vi "Anritsu1a_MT8852B_YYLL_InitialSetting.vi"(11 "YTESTER测试数据":T1) -> (3 "YTESTER结论":T2)   [LabVIEW 2017]
doc: "VIDescription="
uses:
  YtCommon.lvlibp/yt`Step StepBaseInput.ctl
  YtCommon.lvlibp/yt`Step StepResult.ctl
  YtCommon.lvlibp/yt`Step TestData.ctl
  YtCommon.lvlibp/yt`Step System Queue.ctl
  YtCommon.lvlibp
panel:
  out "Show":bool
  out "view send":string
  out "read buffer":string
  in  "YTESTER开放参数":T4={"YTESTER_BaseInput"={"isTest"=TRUE, "isSkip"=FALSE, "StepName"="AnritsuMT8852B初始化", "OnPass"=enum."Next", "OnFail"=enum."Terminate", "ReTestNumber"=0.0}, "VISA resource name"="", "EUT搜索时间[5,60]"=10, "低频线损dB[-40,0]"=-0.1, "中频线损dB[-40,0]"=-0.1, "高频线损dB[-40,0]"=-0.1, "功率输出测试-包类型"=enum."DH1", "单隙灵敏度测试-Tx发射功率dBm[-90,0]"=-70.0, "单隙灵敏度测试-包数量[1,10000]"=600}
  # "initialSetting"
  # "MT8852B"
  # "Anritsu"
  # "YYLL"
  # "MT8852B"
  # "Anritsu"
  # "YYLL"
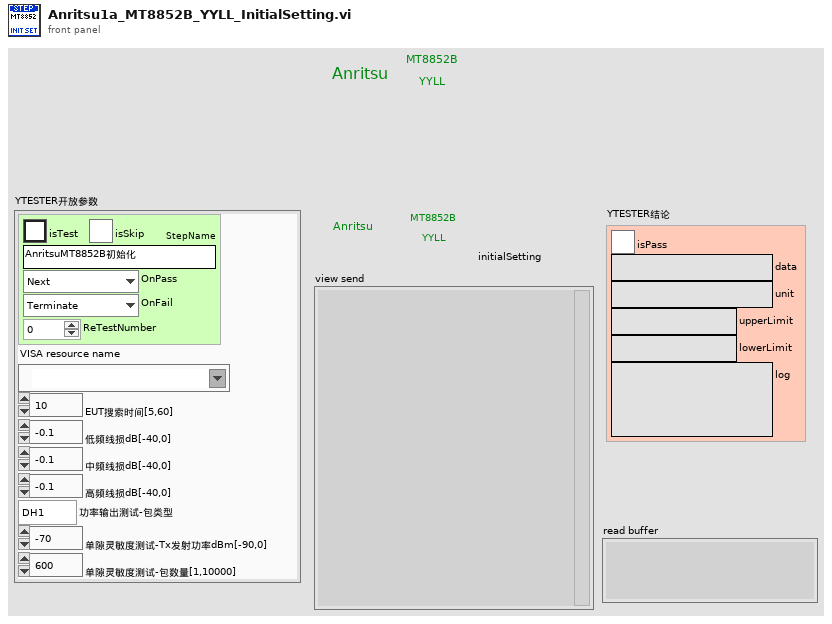
[diagram p1: front panel]
types:
  T1 = typedef "YtCommon.lvlibp/yt`Step TestData.ctl" = cluster{"Socket(From1)":i32, "SN":refnum<notifier>, "StopFlagRef":refnum<notifier>, "YT System Queue":refnum<queue>}
  T2 = typedef "YtCommon.lvlibp/yt`Step StepResult.ctl" = cluster{"isPass":bool, "data":string, "unit":string, "upperLimit":string, "lowerLimit":string, "log":string}
  T3 = typedef "YtCommon.lvlibp/yt`Step StepBaseInput.ctl" = cluster{"isTest":bool, "isSkip":bool, "StepName":string, "OnPass":enum16{"Next", "ToOVER", "Terminate"}, "OnFail":enum16{"Next", "ToOVER", "Terminate"}, "ReTestNumber":dbl}
  T4 = cluster{"YTESTER_BaseInput":T3, "VISA resource name":refnum<visa-resource-name>, "EUT搜索时间[5,60]":u32, "低频线损dB[-40,0]":dbl, "中频线损dB[-40,0]":dbl, "高频线损dB[-40,0]":dbl, "功率输出测试-包类型":enum16{"DH1", "DH3", "DH5", "LONG"}, "单隙灵敏度测试-Tx发射功率dBm[-90,0]":dbl, "单隙灵敏度测试-包数量[1,10000]":u32}
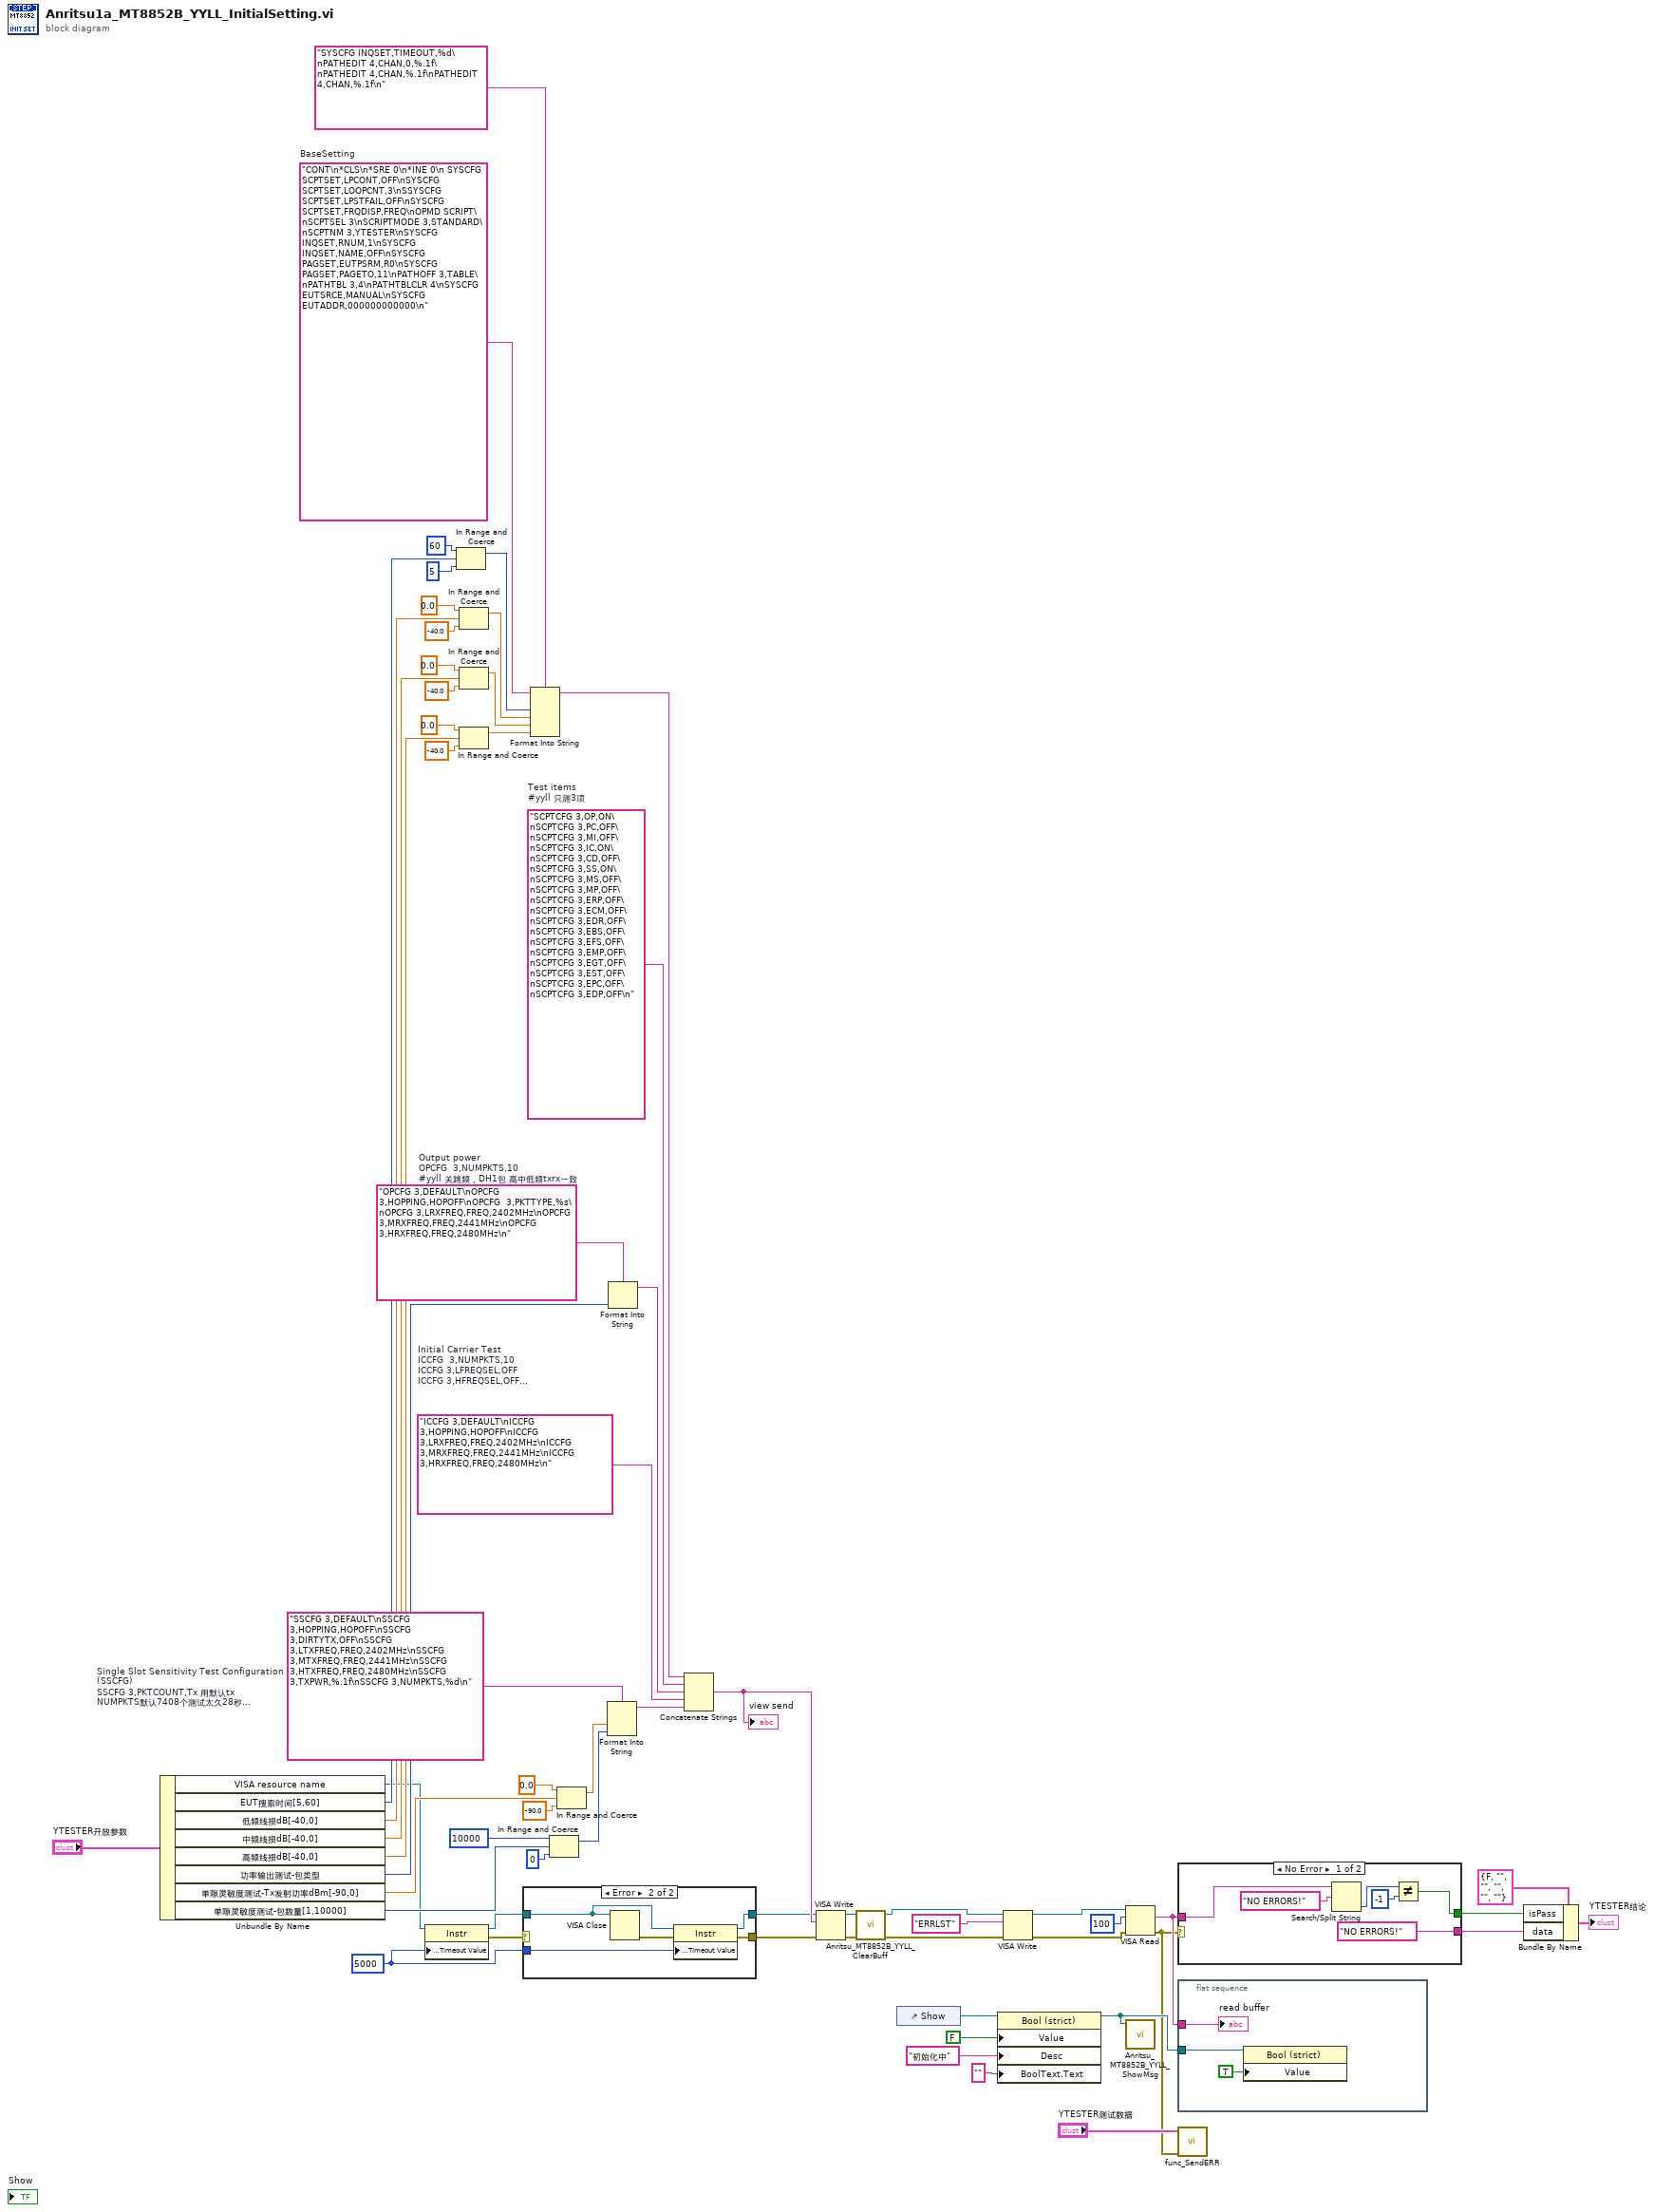
[diagram p0: block diagram]
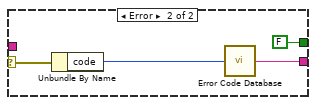
[diagram p3: hidden frame]
diagram:
  w6 = u32 5000 ("General Settings:Timeout Value")
  w21 = "SSCFG 3,DEFAULT\nSSCFG 3,HOPPING,HOPOFF\nSSCFG 3,DIRTYTX,OFF\nSSCFG 3,LTXFREQ,FREQ,2402MHz\nSSCFG 3,MTXFREQ,FREQ,2441MHz\nSSCFG 3,HTXFREQ,FREQ,2480MHz\nSSCFG 3,TXPWR,%.1f\nSSCFG 3,NUMPKTS,%d\n"  # Single Slot Sensitivity Test Configuration (SSCFG)  SSCFG 3,PKTCOUNT,Tx 用默认tx NUMPKTS默认7408个测试太久28秒 控制在600个包吧 #yyll
  w55 = "ICCFG 3,DEFAULT\nICCFG 3,HOPPING,HOPOFF\nICCFG 3,LRXFREQ,FREQ,2402MHz\nICCFG 3,MRXFREQ,FREQ,2441MHz\nICCFG 3,HRXFREQ,FREQ,2480MHz\n"  # Initial Carrier Test  ICCFG  3,NUMPKTS,10 ICCFG 3,LFREQSEL,OFF ICCFG 3,HFREQSEL,OFF #yyll 这里只测中频，关跳频，中频txrx一致 还是都测吧
  w28 = "OPCFG 3,DEFAULT\nOPCFG 3,HOPPING,HOPOFF\nOPCFG  3,PKTTYPE,%s\nOPCFG 3,LRXFREQ,FREQ,2402MHz\nOPCFG 3,MRXFREQ,FREQ,2441MHz\nOPCFG 3,HRXFREQ,FREQ,2480MHz\n"  # Output power OPCFG  3,NUMPKTS,10 #yyll 关跳频，DH1包 高中低频txrx一致
  w60 = "SCPTCFG 3,OP,ON\nSCPTCFG 3,PC,OFF\nSCPTCFG 3,MI,OFF\nSCPTCFG 3,IC,ON\nSCPTCFG 3,CD,OFF\nSCPTCFG 3,SS,ON\nSCPTCFG 3,MS,OFF\nSCPTCFG 3,MP,OFF\nSCPTCFG 3,ERP,OFF\nSCPTCFG 3,ECM,OFF\nSCPTCFG 3,EDR,OFF\nSCPTCFG 3,EBS,OFF\nSCPTCFG 3,EFS,OFF\nSCPTCFG 3,EMP,OFF\nSCPTCFG 3,EGT,OFF\nSCPTCFG 3,EST,OFF\nSCPTCFG 3,EPC,OFF\nSCPTCFG 3,EDP,OFF\n"  # Test items #yyll 只测3项
  w35 = "CONT\n*CLS\n*SRE 0\n*INE 0\n SYSCFG SCPTSET,LPCONT,OFF\nSYSCFG SCPTSET,LOOPCNT,3\nSSYSCFG SCPTSET,LPSTFAIL,OFF\nSYSCFG SCPTSET,FRQDISP,FREQ\nOPMD SCRIPT\nSCPTSEL 3\nSCRIPTMODE 3,STANDARD\nSCPTNM 3,YTESTER\nSYSCFG INQSET,RNUM,1\nSYSCFG INQSET,NAME,OFF\nSYSCFG PAGSET,EUTPSRM,R0\nSYSCFG PAGSET,PAGETO,11\nPATHOFF 3,TABLE\nPATHTBL 3,4\nPATHTBLCLR 4\nSYSCFG EUTSRCE,MANUAL\nSYSCFG EUTADDR,000000000000\n"  # BaseSetting
  n1 = Unbundle By Name("YTESTER开放参数") -> ("VISA resource name"=w5:refnum<visa-resource-name>, "EUT搜索时间[5,60]"=w49:u32, "低频线损dB[-40,0]"=w39:dbl, "中频线损dB[-40,0]"=w38:dbl, "高频线损dB[-40,0]"=w37:dbl, "功率输出测试-包类型"=w30:enum16{"DH1", "DH3", "DH5", "LONG"}, "单隙灵敏度测试-Tx发射功率dBm[-90,0]"=w25:dbl, "单隙灵敏度测试-包数量[1,10000]"=w22:u32)
  n2 = property class="Instr"(reference=w5, "General Settings:Timeout Value"=w6) -> (reference out=w7:refnum<visa-resource-name>, error out=w8:errorcluster)  [unwired: 1 in]
  n3 = In Range and Coerce(upper limit=u32 60, x=w49, lower limit=u32 5) -> (coerced(x)=w46:u32)  [unwired: 1 out]
  n4 = In Range and Coerce(upper limit=0.0, x=w39, lower limit=-40.0) -> (coerced(x)=w34:dbl)  [unwired: 1 out]
  n5 = In Range and Coerce(upper limit=0.0, x=w38, lower limit=-40.0) -> (coerced(x)=w33:dbl)  [unwired: 1 out]
  n6 = In Range and Coerce(upper limit=0.0, x=w37, lower limit=-40.0) -> (coerced(x)=w32:dbl)  [unwired: 1 out]
  n7 = case shown="Error" w8 {
    selector: w8 -> [w63 _]
    tunnel: w7 -> [w64 w69]
    tunnel: w6 -> [_ w67]
    tunnel: [w63 w66] -> w3
    tunnel: [w64 w65] -> w4
    frame No Error {
    }
    frame Error {
      n8 = VISA Close(VISA resource name=w69) -> (error out=w68:errorcluster)  [unwired: 1 in]
      n9 = property class="Instr"(reference=w69, error in=w68, "General Settings:Timeout Value"=w67) -> (reference out=w65:refnum<visa-resource-name>, error out=w66:errorcluster)
    }
  }
  n10 = Format Into String(format string="SYSCFG INQSET,TIMEOUT,%d\nPATHEDIT 4,CHAN,0,%.1f\nPATHEDIT 4,CHAN,%.1f\nPATHEDIT 4,CHAN,%.1f\n", initial string=w35, w46, w34, w33, w32) -> (resulting string=w31:string)  [unwired: 1 in, 1 out]
  n11 = In Range and Coerce(upper limit=u32 10000, x=w22, lower limit=u32 0) -> (coerced(x)=w19:u32)  [unwired: 1 out]
  n12 = In Range and Coerce(upper limit=0.0, x=w25, lower limit=-90.0) -> (coerced(x)=w20:dbl)  [unwired: 1 out]
  n13 = Format Into String(format string=w21, w20, w19) -> (resulting string=w16:string)  [unwired: 2 in, 1 out]
  n14 = Format Into String(format string=w28, w30) -> (resulting string=w29:string)  [unwired: 2 in, 1 out]
  n15 = Concatenate Strings(w31, w60, w29, w55, w16) -> (w17:string)
  "view send" <- w17
  n16 = VISA Write(VISA resource name=w4, write buffer=w17, error in (no error)=w3) -> (VISA resource name out=w54:refnum<visa-resource-name>, error out=w52:errorcluster)  [unwired: 1 out]
  n17 = call "Anritsu_MT8852B_YYLL_ClearBuff.vi"("error IO"=w52, "VISA resource name"=w54) -> ("error IO 2"=w51:errorcluster, "VISA resource name 2"=w53:refnum<visa-resource-name>)  [unwired: 7 in, 1 out]
  n18 = control-ref of="Show"() -> (w15:refnum<vi>)
  n19 = property on="Property Node" class="Bool (strict)"(reference=w15, "Value"=FALSE, "Desc"="初始化中" ("Description"), "BoolText.Text"="" ("Boolean Text.Text")) -> (reference out=w13:refnum<vi>)  [unwired: 1 in, 1 out]
  n20 = VISA Write(VISA resource name=w53, write buffer="ERRLST", error in (no error)=w51) -> (VISA resource name out=w57:refnum<visa-resource-name>, error out=w56:errorcluster)  [unwired: 1 out]
  n21 = VISA Read(VISA resource name=w57, byte count=u32 100 ("byte count (0)"), error in (no error)=w56) -> (read buffer=w12:string, error out=w10:errorcluster)  [unwired: 2 out]
  n22 = call "Anritsu_MT8852B_YYLL_ShowMsg.vi"("reference out"=w13) -> ()  [unwired: 11 in]
  n23 = case shown="No Error" w10 {
    selector: w10 -> [_ w78]
    tunnel: [w71 FALSE] -> w18
    tunnel: w12 -> [w72 _]
    tunnel: ["NO ERRORS!" ("search string/char (-)") w76] -> w9
    frame No Error {
      n24 = Search/Split String(string=w72, search string/char (-)="NO ERRORS!") -> (offset of match=w75:i32)  [unwired: 1 in, 2 out]
      n25 = Not Equal?(x=w75, y=-1) -> (x != y?=w71:bool)
    }
    frame Error {
      n26 = Unbundle By Name(w78) -> ("code"=w77:i32)
      n27 = call <vilib>:"Error Code Database.vi"("Error Code"=w77) -> ("Error Text"=w76:string)
    }
  }
  n28 = flat-sequence {
    tunnel: w13 -> [w81]
    tunnel: w12 -> [w80]
    frame #0 {
      n29 = property on="Property Node" class="Bool (strict)"(reference=w81, "Value"=TRUE) -> ()  [unwired: 1 in, 2 out]
      "read buffer" <- w80
    }
  }
  n30 = call "func_SendERR.vi"("ERR (String\\Errclust)"=w10, "YTESTER测试数据 in"="YTESTER测试数据") -> ()  [unwired: 9 in, 1 out]
  n31 = Bundle By Name(cluster=T2 {"isPass"=FALSE, "data"="", "unit"="", "upperLimit"="", "lowerLimit"="", "log"=""} ("Result"), "isPass"=w18, "data"=w9) -> (→"YTESTER结论":T2)
